vi "dllTest.vi"() -> ()   [LabVIEW 2025]
panel:
  out "Array":string[](array[string])
  out "error":i32
  out "noOfChrIn eacimage":i32[](array[numeric])
  in  "deg":i32=52
  out "before substring":string
  out "x-y":u32
  in  "r":i32=15
  in  "l":i32=15
  out "deviceNum":i32
  out "succ 5":i32
  in  "PathDict":path=path "D:/Test/dllTest/models/en_dict.txt"
  in  "PathModel":path=path "D:/Test/dllTest/models/ocr_model_b1_3x48x480_cuda_16.pt"
  in  "b":i32=80
  in  "t":i32=80
  out "succ 4":i32
  out "succ 3":i32
  out "succ 2":i32
  out "succ":i32
  out "tcv":u64
  out "Image":T1(plugin-control)
  in  "PathImage":path=path "D:/Test/dllTest/images"
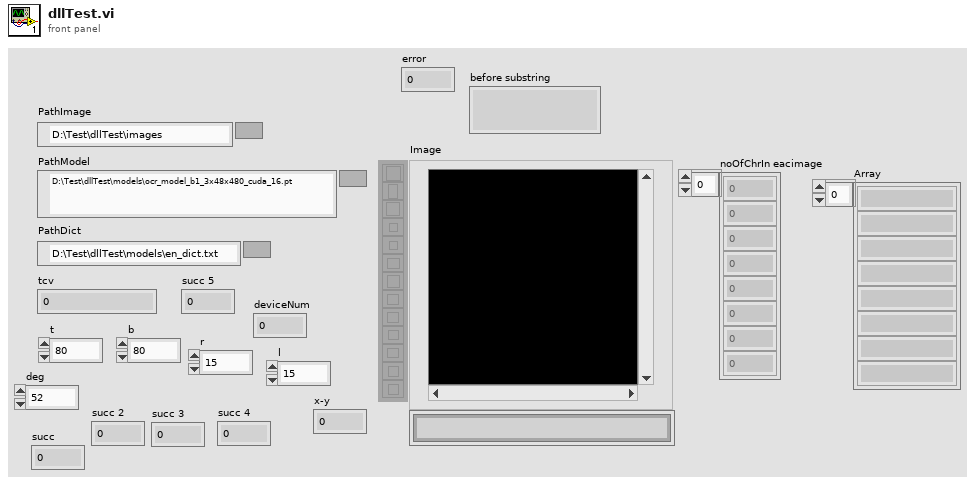
[diagram p1: front panel]
types:
  T1 = typedef "IMAQ Image.ctl" = refnum<image>
  T2 = enum32{"Map Pixel Pointer", "Unmap Pixel Pointer", "Get Pixels Infos"}
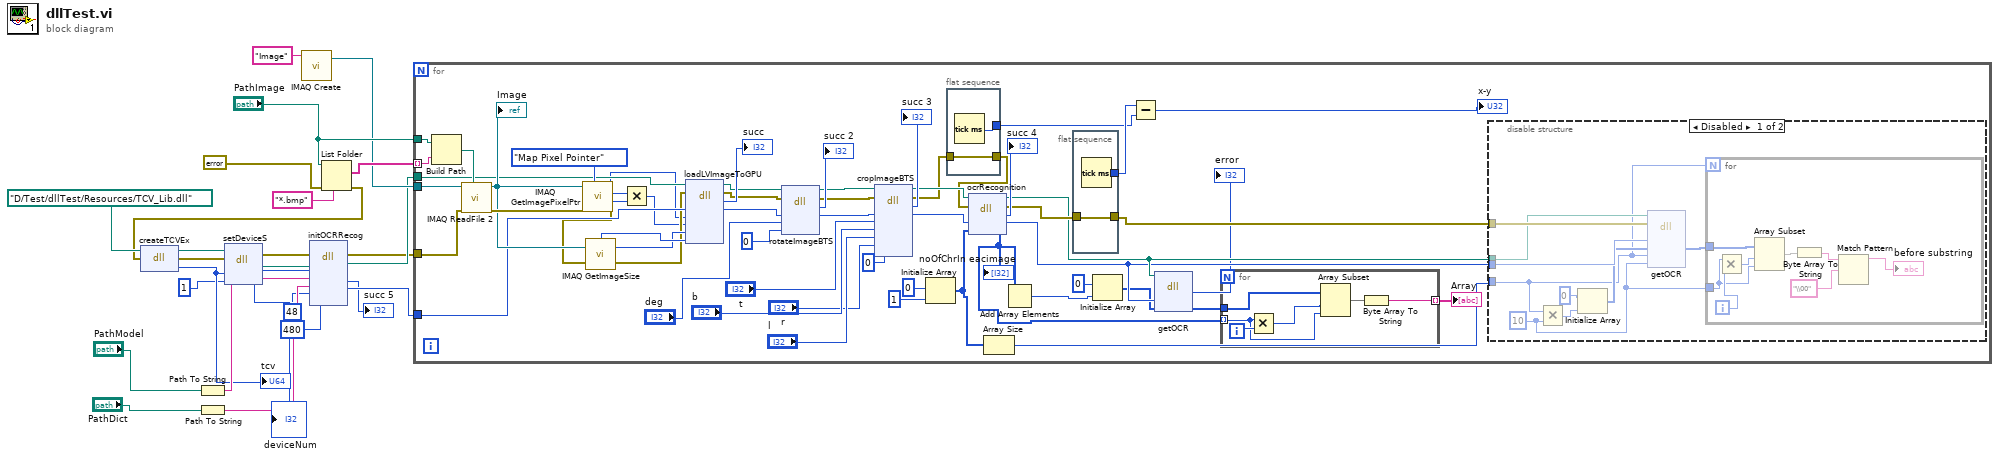
[diagram p0: block diagram]
diagram:
  n1 = Path To String(path="PathModel") -> (string=w15:string)
  n2 = Path To String(path="PathDict") -> (string=w14:string)
  n3 = call "IMAQ Create"("Image Name"="Image") -> ("New Image"=w22:T1)  [unwired: 4 in, 1 out]
  n4 = List Folder(path="PathImage", pattern="*.bmp", error in=errorcluster {"status"=FALSE, "code"=0, "source"=""}) -> (filenames=w24:string[], error out=w19:errorcluster)  [unwired: 1 in, 2 out]
  n5 = dll-call lib="D:/Test/dllTest/Resources/TCV_Lib.dll" fn="createTCVEx"(path in=path "D:/Test/dllTest/Resources/TCV_Lib.dll", error in=w19) -> (path out=w8:path, error out=w7:errorcluster, "tcv"=w6:u64)  [unwired: 1 in]
  "tcv" <- w6
  n6 = dll-call lib="D:/Test/dllTest/Resources/TCV_Lib.dll" fn="setDeviceS"(path in=w8, error in=w7, "TCV"=w6, "device"=1) -> (path out=w4:path, error out=w3:errorcluster, "deviceNum"=→"deviceNum":i32, "TCV"=w2:u64)  [unwired: 2 in]
  n7 = dll-call lib="D:/Test/dllTest/Resources/TCV_Lib.dll" fn="initOCRRecog"(path in=w4, error in=w3, "TCV"=w2, "modelPath"=w15, "dictPath"=w14, "height"=48, "width"=480) -> (path out=w18:path, error out=w17:errorcluster, "succ"=→"succ 5":i32, "TCV"=w16:u64)  [unwired: 5 in]
  n8 = for {
    tunnel: "PathImage" -> [w83]
    tunnel: w24 -> [w82] mode=indexing
    tunnel: w22 -> [w80]
    tunnel: w16 -> [w74]
    tunnel: w18 -> [w73]
    tunnel: w17 -> [w50]
    n9 = Build Path(base path=w83, name or relative path=w82) -> (appended path=w81:path)
    n10 = call "IMAQ ReadFile 2"("File Path"=w81, "error in (no error)"=w50, "Image"=w80) -> ("error out"=w79:errorcluster, "Image Out"=w77:T1)  [unwired: 4 in, 3 out]
    "Image" <- w77
    n11 = call "IMAQ GetImagePixelPtr"("Function"=T2."Map Pixel Pointer", "error in (no error)"=w79, "Image"=w77) -> ("error out"=w71:errorcluster, "Pixel Size (Bytes)"=w69:i32, "LineWidth(Pixels)"=w70:i32, "Pixel Pointer out"=w67:u64)  [unwired: 3 in, 2 out]
    n12 = call "IMAQ GetImageSize"("Image"=w77, "error in (no error)"=w71) -> ("Y Resolution"=w75:i32, "X Resolution"=w76:i32, "error out"=w72:errorcluster)  [unwired: 2 in]
    n13 = Multiply(x=w70, y=w69) -> (x*y=w68:i32)
    n14 = dll-call lib="D:/Test/dllTest/Resources/TCV_Lib.dll" fn="loadLVImageToGPU"(path in=w73, error in=w72, "tcv"=w74, "imgPtr"=w67, "lw"=w68, "h"=w75, "w"=w76) -> (path out=w65:path, error out=w64:errorcluster, "succ"=→"succ":i32, "tcv"=w63:u64)  [unwired: 5 in]
    n15 = dll-call lib="D:/Test/dllTest/Resources/TCV_Lib.dll" fn="rotateImageBTS"(path in=w65, error in=w64, "TCV"=w63, "deg"="deg", "show"=0) -> (path out=w60:path, error out=w59:errorcluster, "succ"=→"succ 2":i32, "TCV"=w58:u64)  [unwired: 3 in]
    n16 = dll-call lib="D:/Test/dllTest/Resources/TCV_Lib.dll" fn="cropImageBTS"(path in=w60, error in=w59, "TCV"=w58, "t"="t", "b"="b", "l"="l", "r"="r", "show"=0) -> (path out=w55:path, error out=w45:errorcluster, "succ"=→"succ 3":i32, "TCV"=w54:u64)  [unwired: 6 in]
    n17 = Initialize Array(0 ("batch"), 1 ("dimension size")) -> (w30:i32[])
    n18 = flat-sequence {
      tunnel: w45 -> [w110]
      tunnel: [w110] -> w44
      tunnel: [w109] -> w42
      frame #0 {
        n19 = Tick Count (ms)() -> (millisecond timer value=w109:u32)
      }
    }
    n20 = dll-call lib="D:/Test/dllTest/Resources/TCV_Lib.dll" fn="ocrRecognition"(path in=w55, error in=w44, "TCV"=w54, "noOfChrIn eacimage"=w30) -> (path out=w34:path, error out=w46:errorcluster, "succ"=→"succ 4":i32, "TCV"=w33:u64, "noOfChrIn eacimage"=w28:i32[])  [unwired: 1 in]
    "noOfChrIn eacimage" <- w28
    n21 = Array Size(array=w30) -> (size(s)=w37:i32)
    n22 = Add Array Elements(numeric array=w28) -> (sum=w35:i32)
    n23 = flat-sequence {
      tunnel: w46 -> [w108]
      tunnel: [w108] -> w40
      tunnel: [w107] -> w43
      frame #0 {
        n24 = Tick Count (ms)() -> (millisecond timer value=w107:u32)
      }
    }
    n25 = Initialize Array(u8 0 ("element"), w35) -> (w32:u8[])
    n26 = Subtract(x=w43, y=w42) -> (x-y=→"x-y":u32)
    n27 = dll-call lib="D:/Test/dllTest/Resources/TCV_Lib.dll" fn="getOCR"(path in=w34, "TCV"=w33, "buffer"=w32) -> ("error"=→"error":i32, "buffer"=w31:u8[])  [unwired: 3 in, 2 out]
    n28 = for {
      tunnel: w31 -> [w89]
      tunnel: w28 -> [w86] mode=indexing
      tunnel: [w84] -> w27 mode=indexing
      i -> [w88]
      n29 = Multiply(x=w86, y=w88) -> (x*y=w87:i32)
      n30 = Array Subset(array=w89, index=w87, length=w86) -> (w85:u8[])
      n31 = Byte Array To String(unsigned byte array=w85) -> (string=w84:string)
    }
    "Array" <- w27
    n32 = disable-structure shown="Disabled" {
      disable-tunnel: w40 -> [w98 _]
      disable-tunnel: w34 -> [w97 _]
      disable-tunnel: w33 -> [w96 _]
      disable-tunnel: w37 -> [w92 _]
      frame Disabled {
        w90 = 10 ("y")
        n33 = Multiply(x=w92, y=w90) -> (x*y=w95:i32)
        n34 = Initialize Array(u8 0 ("element"), w95) -> (w93:u8[])
        n35 = dll-call lib="D:/Test/dllTest/Resources/TCV_Lib.dll" fn="getOCR"(path in=w97, error in=w98, "TCV"=w96, "arr"=w93, "numStrings"=w92, "maxLen"=w90) -> ("arr"=w91:u8[])  [unwired: 5 in, 2 out]
        n36 = for {
          N: w92 -> [_]
          tunnel: w91 -> [w106]
          tunnel: w90 -> [w99]
          i -> [w105]
          n37 = Multiply(x=w99, y=w105) -> (x*y=w100:i32)
          n38 = Array Subset(array=w106, index=w100, length=w99) -> (w104:u8[])
          n39 = Byte Array To String(unsigned byte array=w104) -> (string=w103:string)
          n40 = Match Pattern(string=w103, regular expression="\\00") -> (before substring=→"before substring":string)  [unwired: 1 in, 3 out]
        }
      }
      frame Enabled {
      }
    }
  }
